vi "Read value.vi"(8 "error in (no error)":errorcluster, 11 "id in":refnum<class "id.lvclass">) -> (0 "error out":errorcluster, 2 "value":string, 3 "id out":refnum<class "id.lvclass">)   [LabVIEW 2015, in "id.lvclass"]
uses:
  id.lvclass
  JSONable/JSONable.lvclass
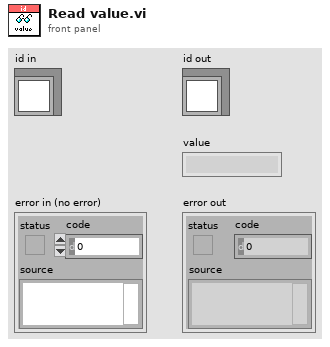
[diagram p1: front panel]
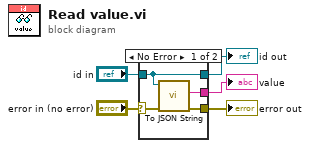
[diagram p0: block diagram]
diagram:
  n1 = case shown="No Error" "error in (no error)" {
    selector: "error in (no error)" -> [w7 w10]
    tunnel: [w6 w10] -> w4
    tunnel: [w9 w11] -> w2
    tunnel: "id in" -> [w9 w11]
    tunnel: [w8 _] -> w1
    frame No Error {
      n2 = call "To JSON String.vi"("error in (no error)"=w7, "JSONable in"=w9) -> ("error out"=w6:errorcluster, "JSON String"=w8:string)  [unwired: 7 in, 1 out]
    }
    frame Error {
    }
  }
  "error out" <- w4
  "id out" <- w2
  "value" <- w1
